vi "Get Sentence Type.vi"(8 "error in (no error)":errorcluster, 11 "sentence":string) -> (0 "error out":errorcluster, 1 "valid sentence?":bool, 3 "sentence type":string)   [LabVIEW 2017, in "NMEA API.lvlib"]
doc: "Returns the type of an NMEA <B>sentence</B>. The first token following $ in an NMEA sentence is the <B>sentence type</B>. The type of a sentence defines the contents and interpretation of the sentence."
uses:
  <vilib>/robotics/Protocols/NMEA/NMEA API.lvlib
  <vilib>/regexp/Match Regular Expression.xnode
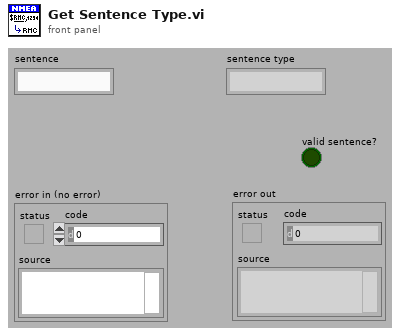
[diagram p1: front panel]
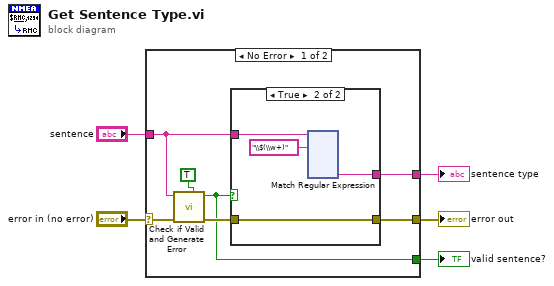
[diagram p0: block diagram]
diagram:
  n1 = case shown="No Error" "error in (no error)" {
    selector: "error in (no error)" -> [w10 w131]
    tunnel: [w11 w131] -> w5
    tunnel: [w12 _] -> w4
    tunnel: "sentence" -> [w8 _]
    tunnel: [w7 _] -> w1
    frame No Error {
      n2 = call <vilib>:"Check if Valid and Generate Error.vi"("generate error if invalid (F)"=TRUE, "error in (no error)"=w10, "sentence"=w8) -> ("error out"=w9:errorcluster, "valid sentence"=w7:bool)  [unwired: 7 in]
      n3 = case shown="True" w7 {
        tunnel: [_ w16] -> w12
        tunnel: [w13 w15] -> w11
        tunnel: w9 -> [w13 w15]
        tunnel: w8 -> [_ w14]
        frame False {
          # "Invalid sentence"
        }
        frame True {
          n4 = xnode "Match Regular Expression"("input string"=w14, "regular expression"="\\$(\\w+)") -> ("submatch 1"=w16:string)  [unwired: 2 in, 7 out]
        }
      }
    }
    frame Error {
      # "If there is an error coming in,\nthen it just returns that error\nand an empty string"
    }
  }
  "sentence type" <- w4
  "error out" <- w5
  "valid sentence?" <- w1
